vi "SelectChosenPoints.vi"(2 "error in (no error)":errorcluster, 3 "Points array":cluster{"Edge Info":T1, "Boolean":bool}[](array[cluster]) {"Edge Info"."Distance (Real-World)" format="%.2f"; "Edge Info"."Location (Real-World)"."Y" format="%.2g"; "Edge Info"."Location (Real-World)"."X" format="%.2f"; "Edge Info"."Noise" format="%.2f"; "Edge Info"."Location (Pixel)"."Y" format="%.2g"; "Edge Info"."Location (Pixel)"."X" format="%.2f"; "Edge Info"."Strength" format="%.2f"; "Edge Info"."Distance (Pixel)" format="%.2f"}) -> (0 "error out":errorcluster, 1 "array":cluster{"X":sgl, "Y":sgl}[](array[cluster]))   [LabVIEW 2015]
uses:
  <vilib>/vision/Measure.llb/Edge New.ctl
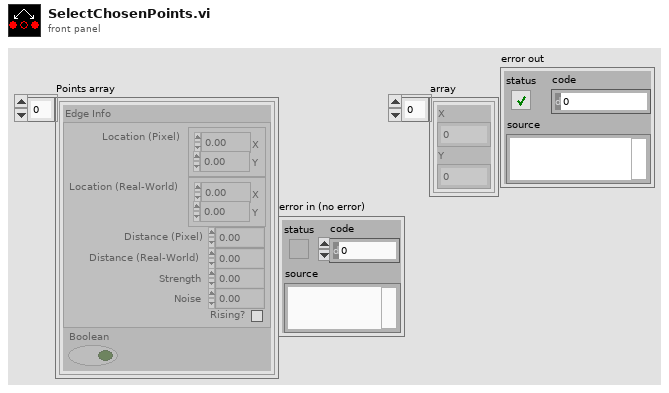
[diagram p1: front panel]
types:
  T1 = typedef "Edge New.ctl" = cluster{"Location (Pixel)":cluster{"X":sgl, "Y":sgl}, "Location (Real-World)":cluster{"X":sgl, "Y":sgl}, "Distance (Pixel)":dbl, "Distance (Real-World)":dbl, "Strength":dbl, "Noise":dbl, "Rising?":bool}
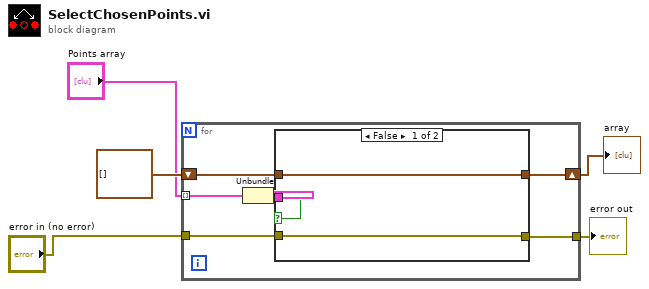
[diagram p0: block diagram]
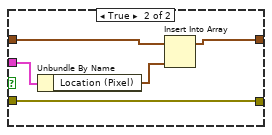
[diagram p2: hidden frame]
diagram:
  n1 = for {
    tunnel: "Points array" -> [w12] mode=indexing
    shift-right: [w9] -> w5
    shift-left: cluster{"X":sgl, "Y":sgl}[] [] ("array") -> [w8]
    tunnel: "error in (no error)" -> [w7]
    tunnel: [w6] -> w1
    n2 = Unbundle(w12) -> ("Edge Info"=w11:T1, "Boolean"=w10:bool)
    n3 = case shown="False" w10 {
      tunnel: w11 -> [_ w19]
      tunnel: [w14 w17] -> w9
      tunnel: w8 -> [w14 w16]
      tunnel: w7 -> [w13 w15]
      tunnel: [w13 w15] -> w6
      frame False {
      }
      frame True {
        n4 = Unbundle By Name(w19) -> ("Location (Pixel)"=w18:cluster{"X":sgl, "Y":sgl})
        n5 = Insert Into Array(array=w16, new element=w18) -> (w17:cluster{"X":sgl, "Y":sgl}[])  [unwired: 1 in]
      }
    }
  }
  "array" <- w5
  "error out" <- w1
